vi "TDC_getHbtParams.vi"(8 "Error In":errorcluster) -> (0 "Error Out":errorcluster, 2 "Bin Count":i32=100, 3 "Bin width [ps]":i32=2)   [LabVIEW 2011]
uses:
  tdcbase.dll
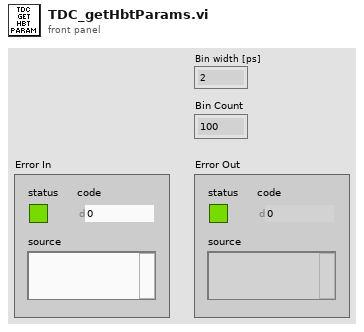
[diagram p1: front panel]
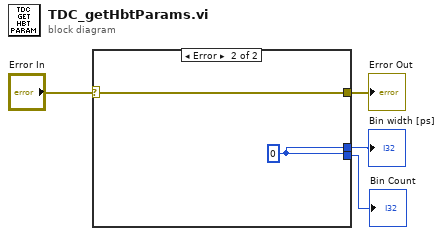
[diagram p0: block diagram]
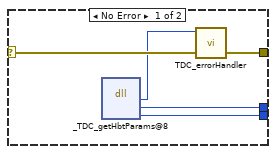
[diagram p2: hidden frame]
diagram:
  n1 = case shown="Error" "Error In" {
    selector: "Error In" -> [w9 w11]
    tunnel: [w8 w11] -> w3
    tunnel: [w6 w10] -> w2
    tunnel: [w5 w10] -> w1
    frame No Error {
      n2 = dll-call lib="X:/tdcbase.dll" fn="_TDC_getHbtParams@8"() -> ("return type"=w7:i32, "binWidth"=w6:i32, "binCount"=w5:i32)  [unwired: 5 in, 2 out]
      n3 = call "TDC_errorHandler.vi"("Error In"=w9, "TDC Return Code"=w7) -> ("Error Out"=w8:errorcluster)  [unwired: 9 in]
    }
    frame Error {
      w10 = 0
    }
  }
  "Error Out" <- w3
  "Bin width [ps]" <- w2
  "Bin Count" <- w1
